vi "Error-Offset.vi"() -> (0 "Error Offset":i32)   [LabVIEW 2018, in "Scripting.lvlib"]
uses:
  Scripting.lvlib
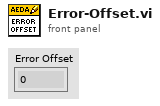
[diagram p1: front panel]
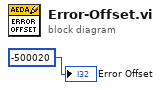
[diagram p0: block diagram]
diagram:
  "Error Offset" <- -500020
